vi "addNewChannelData.vi"(6 "Data In":T1={"Timestamps ms"=[0.0, 0.005, 0.009, 0.012], "DataPerChannel"=[]} {"Timestamps ms" format="%.3f"}, 8 "error in (no error)":errorcluster, 9 "fill number":i32[](array[numeric]), 10 "position":i32[](array[numeric]), 11 "DIO64Output in":refnum<class "DIO64Output.lvclass">) -> (0 "error out":errorcluster, 2 "Dataout":T1, 3 "DIO64Output out":refnum<class "DIO64Output.lvclass">)   [LabVIEW 2011, in "Hardware.lvlib" / "Channels.lvlib" / "DIO64Output.lvclass"]
uses:
  DIO64Output.lvclass
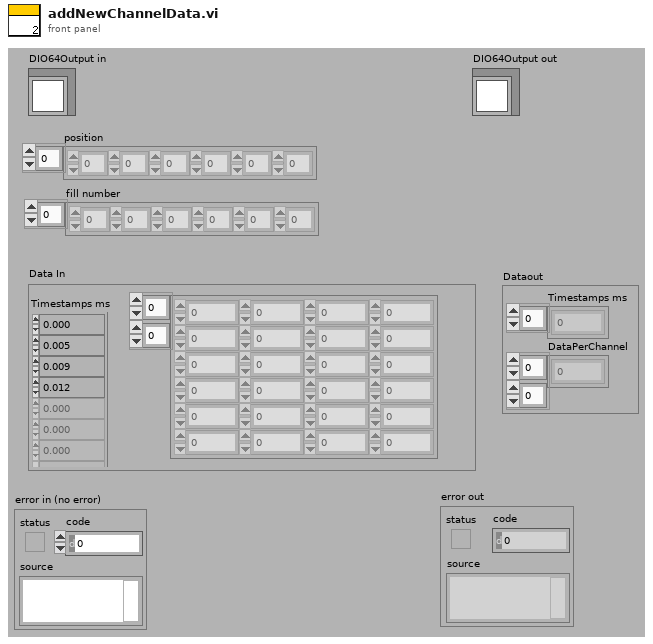
[diagram p1: front panel]
types:
  T1 = cluster{"Timestamps ms":dbl[], "DataPerChannel":dbl[][]}
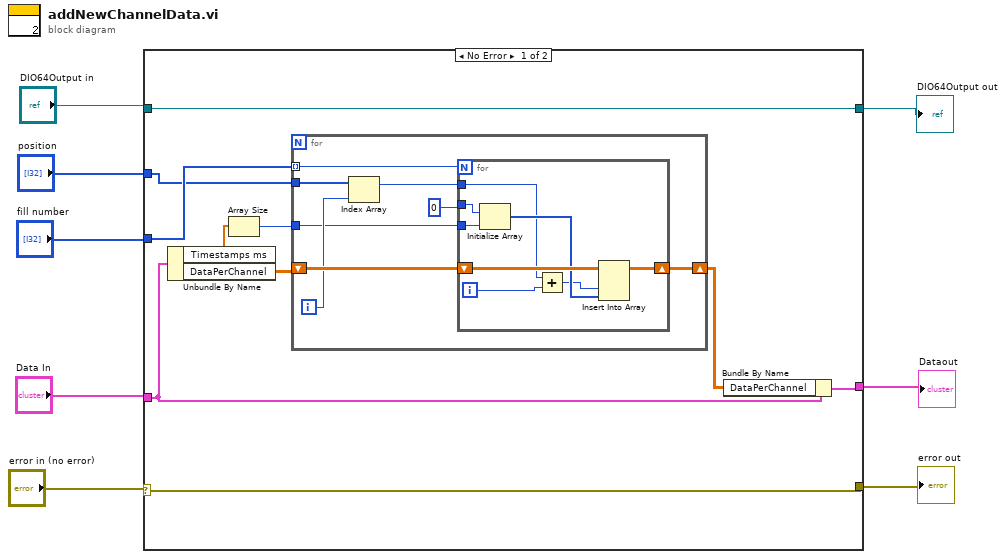
[diagram p0: block diagram]
diagram:
  n1 = case shown="No Error" "error in (no error)" {
    selector: "error in (no error)" -> [w9 w36]
    tunnel: [w9 w36] -> w7
    tunnel: [w15 w35] -> w5
    tunnel: "DIO64Output in" -> [w15 w35]
    tunnel: "position" -> [w17 _]
    tunnel: "fill number" -> [w18 _]
    tunnel: "Data In" -> [w11 _]
    tunnel: [w10 _] -> w1
    frame No Error {
      n2 = Unbundle By Name(w11) -> ("Timestamps ms"=w16:dbl[], "DataPerChannel"=w13:dbl[][])
      n3 = Array Size(array=w16) -> (size(s)=w14:i32)
      n4 = for {
        tunnel: w18 -> [w23] mode=indexing
        shift-right: [w24] -> w12
        shift-left: w13 -> [w25]
        tunnel: w17 -> [w22]
        tunnel: w14 -> [w19]
        i -> [w21]
        n5 = Index Array(array=w22, index=w21) -> (element=w20:i32)
        n6 = for {
          N: w23 -> [_]
          tunnel: 0 -> [w34]
          shift-right: [w31] -> w24
          shift-left: w25 -> [w33]
          tunnel: w20 -> [w29]
          tunnel: w19 -> [w27]
          i -> [w30]
          n7 = Initialize Array(w34, w27) -> (w32:i32[])
          n8 = Add(x=w29, y=w30) -> (x+y=w28:i32)
          n9 = Insert Into Array(array=w33, index (col)=w28, new element=w32) -> (w31:dbl[][])  [unwired: 1 in]
        }
      }
      n10 = Bundle By Name(cluster=w11, "DataPerChannel"=w12) -> (w10:T1)
    }
    frame Error {
    }
  }
  "error out" <- w7
  "DIO64Output out" <- w5
  "Dataout" <- w1
